vi "Read VI to Place Engines and IO Nodes.vi"(8 "error in (no error)":errorcluster, 11 "RIO Target Configuration in":refnum<class "RIO Target Configuration.lvclass">) -> (0 "error out":errorcluster, 2 "VI to Place Engines and IO Nodes":path, 3 "RIO Target Configuration out":refnum<class "RIO Target Configuration.lvclass">)   [LabVIEW 2014, in "RIO Target Configuration.lvclass"]
uses:
  RIO Target Configuration.lvclass
  <vilib>/NI/Configuration Framework/serializable configuration/NISE_CEF_serializable configuration.lvclass
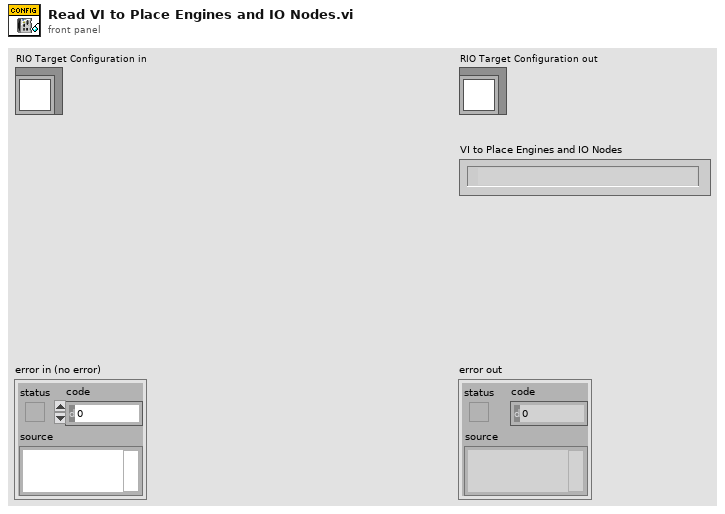
[diagram p1: front panel]
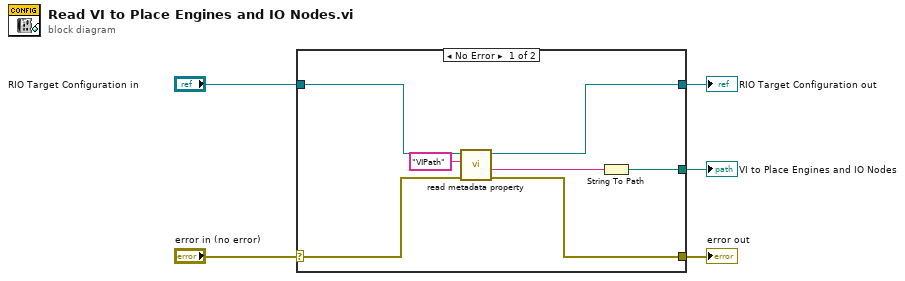
[diagram p0: block diagram]
diagram:
  n1 = case shown="No Error" "error in (no error)" {
    selector: "error in (no error)" -> [w10 w13]
    tunnel: [w9 w13] -> w4
    tunnel: [w11 w14] -> w2
    tunnel: "RIO Target Configuration in" -> [w12 w14]
    tunnel: [w7 _] -> w1
    frame No Error {
      n2 = call <vilib>:"read metadata property.vi"("error in"=w10, "key"="VIPath", "configuration in"=w12) -> ("error out"=w9:errorcluster, "value"=w8:string, "configuration out"=w11:refnum<class "RIO Target Configuration.lvclass">)  [unwired: 5 in, 1 out]
      n3 = String To Path(string=w8) -> (path=w7:path)
    }
    frame Error {
    }
  }
  "error out" <- w4
  "RIO Target Configuration out" <- w2
  "VI to Place Engines and IO Nodes" <- w1
